vi "run.vi"() -> ()   [LabVIEW 2014]
uses:
  creeper.ctl
  nail.ctl
  block.ctl
  airplane.ctl
  <vilib>/Utility/miscctls.llb/LVPositionTypeDef.ctl
  <vilib>/Utility/inputDevices.llb/keyboardAcquire.vi
panel:
  out "step":u32
  in  "airplane":T1
  in  "Block":T2
  in  "nail":T3
  in  "creeper":T4
  out "speed":u32
  out "score":u32
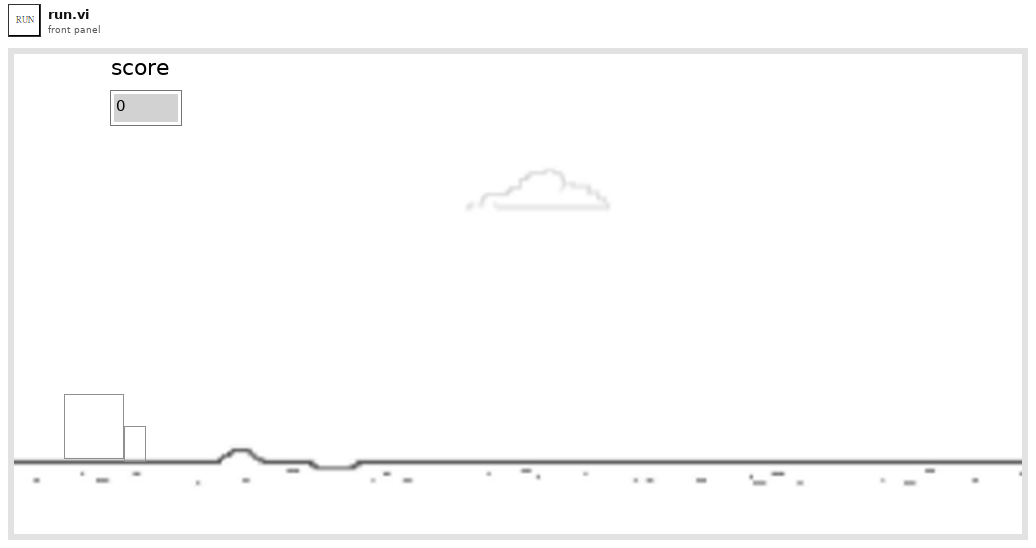
[diagram p1: front panel]
types:
  T1 = typedef "airplane.ctl" = bool
  T2 = typedef "block.ctl" = bool
  T3 = typedef "nail.ctl" = bool
  T4 = typedef "creeper.ctl" = bool
  T5 = typedef "LVPositionTypeDef.ctl" = cluster{"Left":i32, "Top":i32}
  T6 = enum16{"0", "1", "2", "3", "4", "5", "6", "7", "8", "9", "A", "B", "C", "D", "E", "F", "G", "H", "I", "J", "K", "L", "M", "N", "O", "P", "Q", "R", "S", "T", "U", "V", "W", "X", "Y", "Z", "F1", "F2", "F3", "F4", "F5", "F6", "F7", "F8", "F9", "F10", "F11", "F12", "F13", "F14", "F15", "ADD", "BACK", "BACKSLASH", "CAPITAL", "COMMA", "DECIMAL", "DELETE", "DIVIDE", "DOWN", "END", "EQUALS", "ESCAPE", "GRAVE (`)", "HOME", "INSERT", "LBRACKET", "LCONTROL", "LEFT", "L ALT", "LSHIFT", "LWIN", "MINUS", "MULTIPLY", "NEXT", "NUMLOCK", "NUMPAD_0", "NUMPAD_1", "NUMPAD_2", "NUMPAD_3", "NUMPAD_4", "NUMPAD_5", "NUMPAD_6", "NUMPAD_7", "NUMPAD_8", "NUMPAD_9", "PAUSE", "PERIOD", "PRIOR (PG UP)", "RBRACKET", "RCONTROL", "RETURN", "RIGHT", "R ALT", "RSHIFT", "RWIN", "SCROLL", "SEMICOLON", "SLASH", "SPACE", "SUBTRACT", "TAB", "UP", "ENTER (num pad)", "' (quote)"}[]
  T7 = enum16{"0", "1", "2", "3", "4", "5", "6", "7", "8", "9", "A", "B", "C", "D", "E", "F", "G", "H", "I", "J", "K", "L", "M", "N", "O", "P", "Q", "R", "S", "T", "U", "V", "W", "X", "Y", "Z", "F1", "F2", "F3", "F4", "F5", "F6", "F7", "F8", "F9", "F10", "F11", "F12", "F13", "F14", "F15", "ADD", "BACK", "BACKSLASH", "CAPITAL", "COMMA", "DECIMAL", "DELETE", "DIVIDE", "DOWN", "END", "EQUALS", "ESCAPE", "GRAVE (`)", "HOME", "INSERT", "LBRACKET", "LCONTROL", "LEFT", "L ALT", "LSHIFT", "LWIN", "MINUS", "MULTIPLY", "NEXT", "NUMLOCK", "NUMPAD_0", "NUMPAD_1", "NUMPAD_2", "NUMPAD_3", "NUMPAD_4", "NUMPAD_5", "NUMPAD_6", "NUMPAD_7", "NUMPAD_8", "NUMPAD_9", "PAUSE", "PERIOD", "PRIOR (PG UP)", "RBRACKET", "RCONTROL", "RETURN", "RIGHT", "R ALT", "RSHIFT", "RWIN", "SCROLL", "SEMICOLON", "SLASH", "SPACE", "SUBTRACT", "TAB", "UP", "ENTER (num pad)", "' (quote)"}
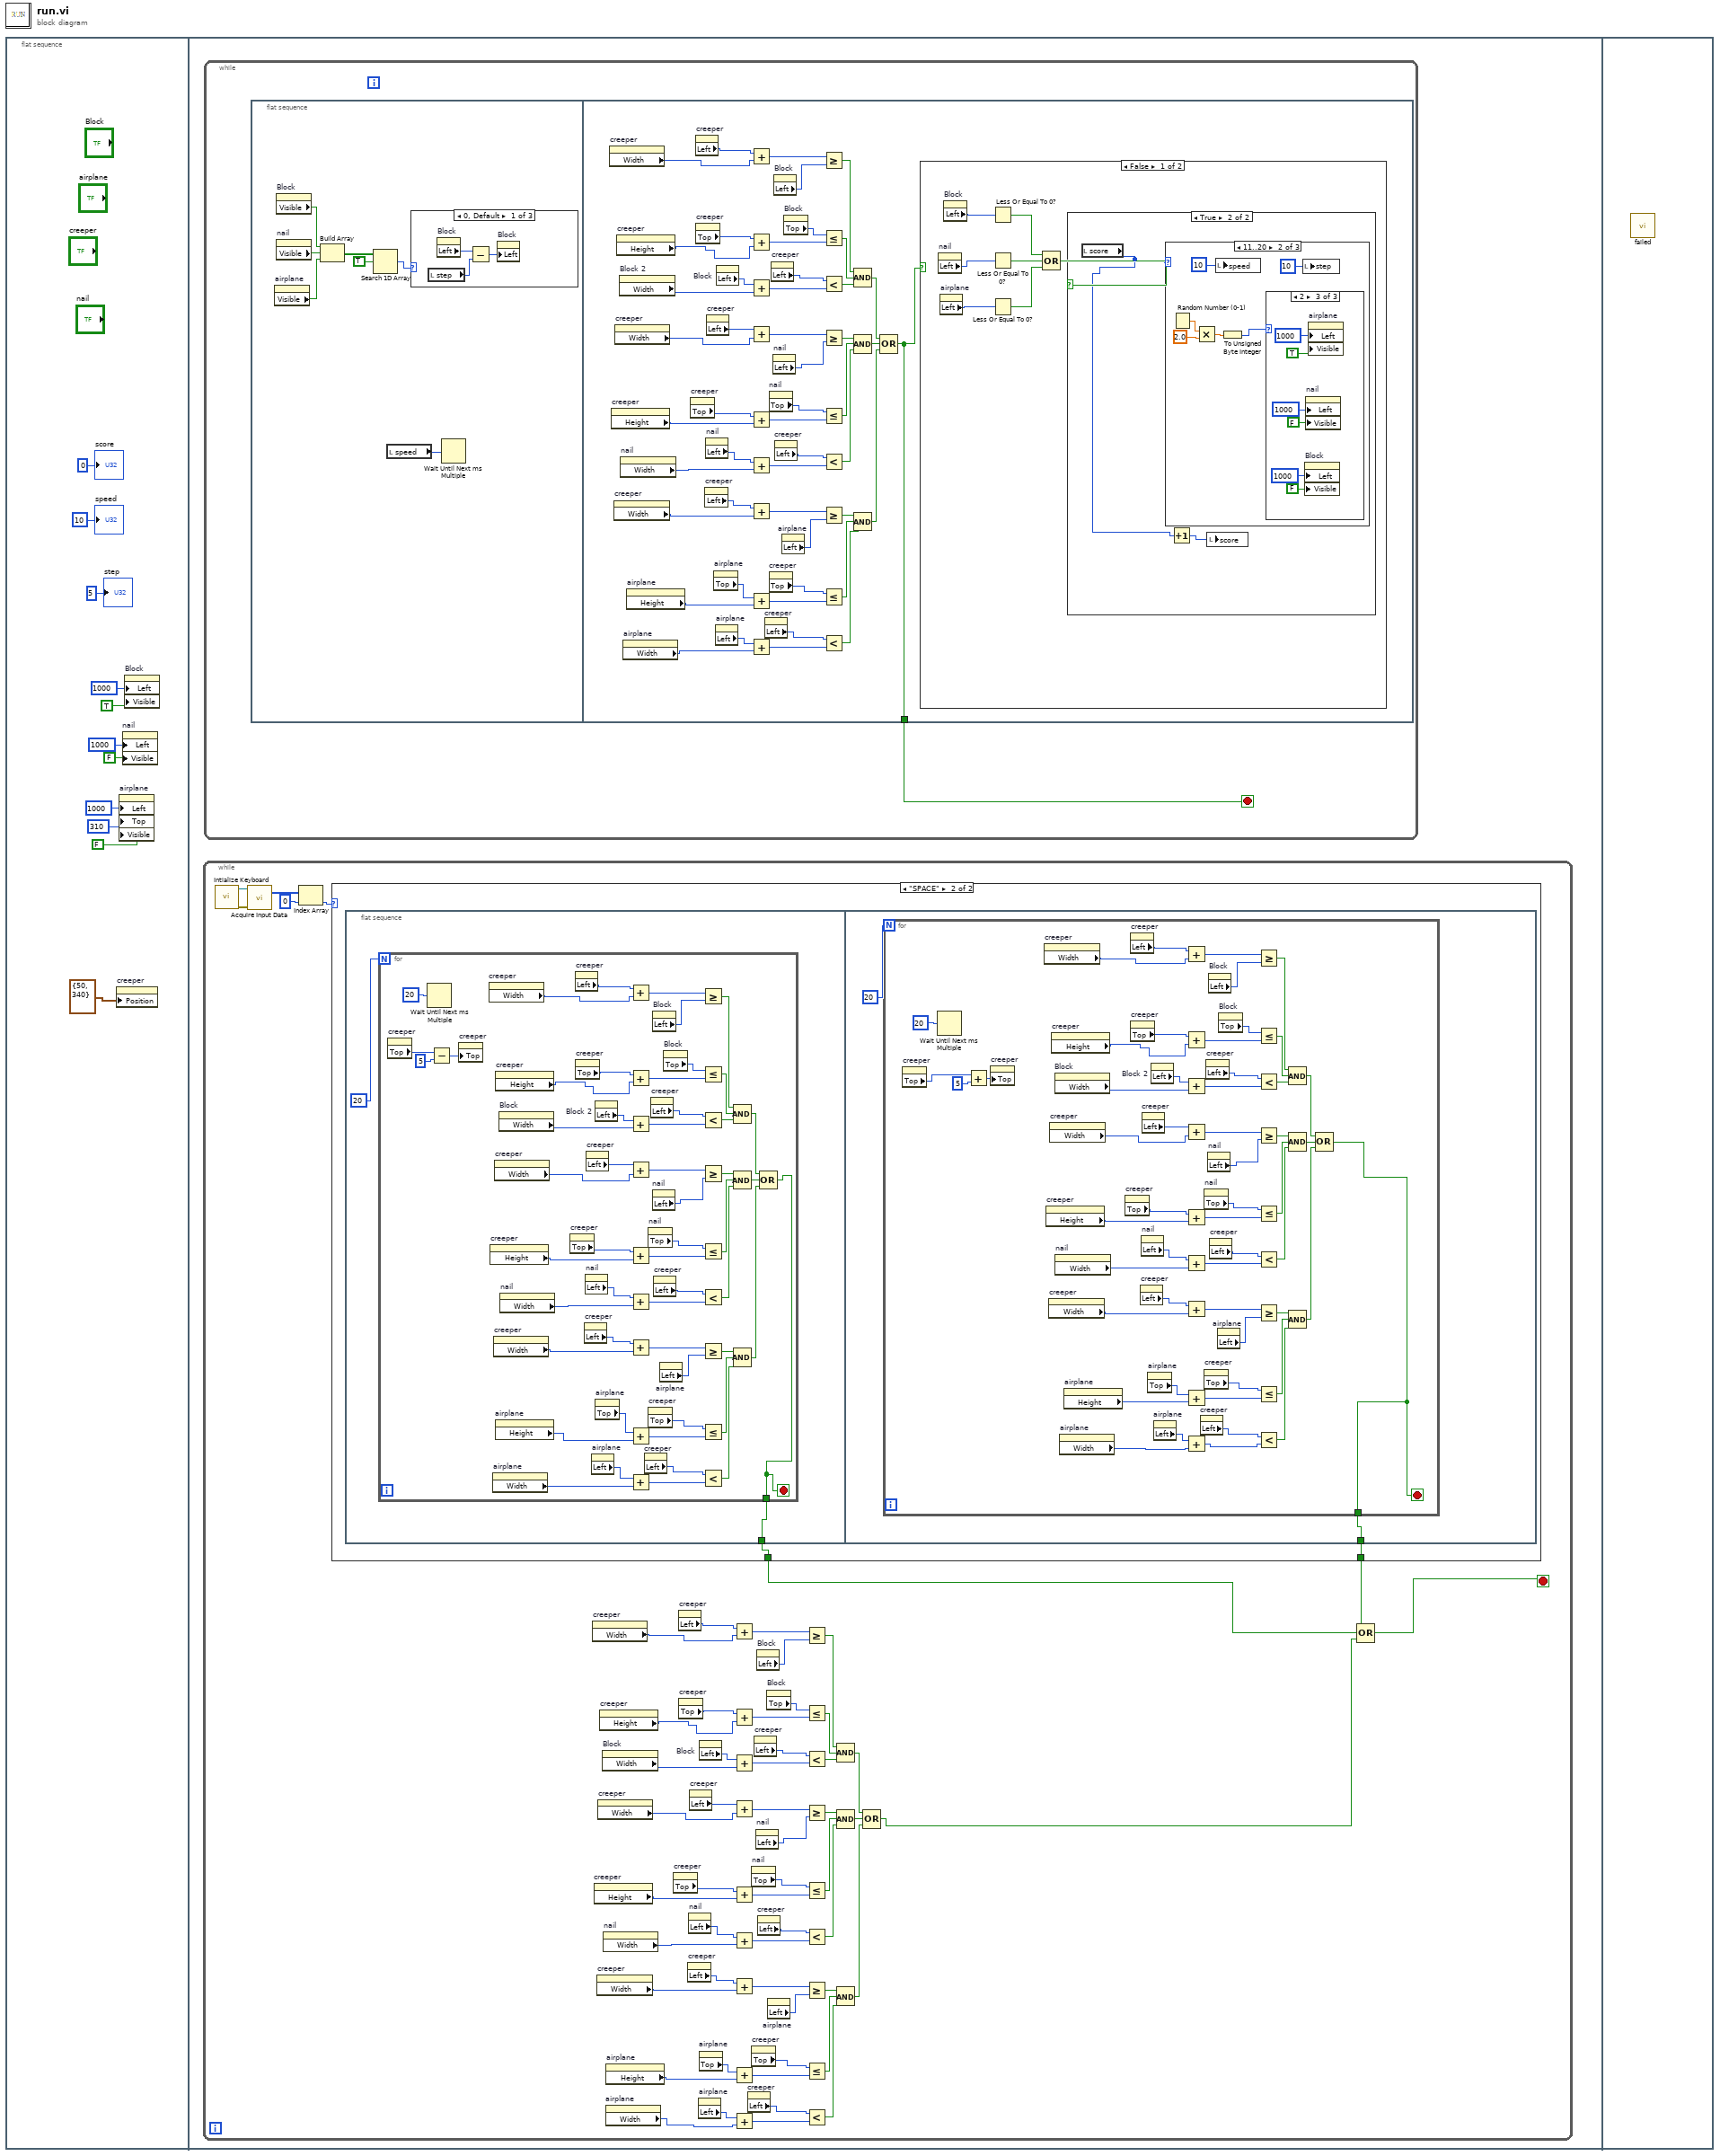
[diagram p0: block diagram]
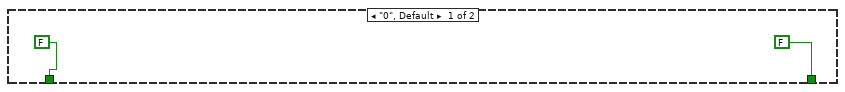
[diagram p2: hidden frame]
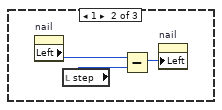
[diagram p3: hidden frame]
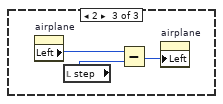
[diagram p4: hidden frame]
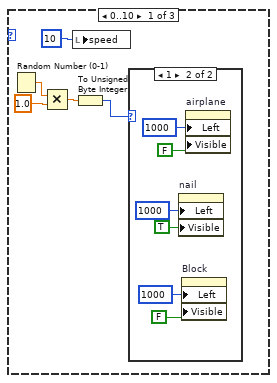
[diagram p6: hidden frame]
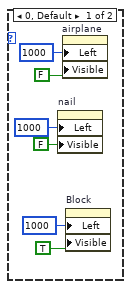
[diagram p7: hidden frame]
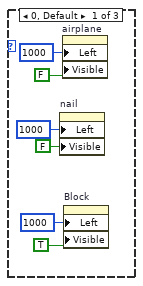
[diagram p8: hidden frame]
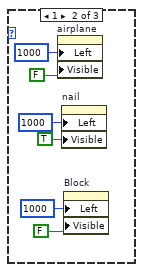
[diagram p9: hidden frame]
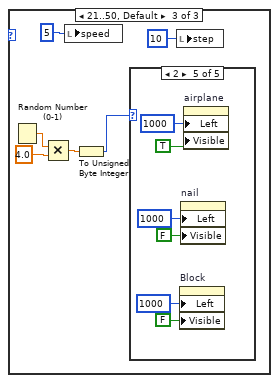
[diagram p10: hidden frame]
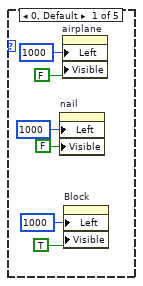
[diagram p11: hidden frame]
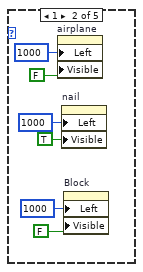
[diagram p12: hidden frame]
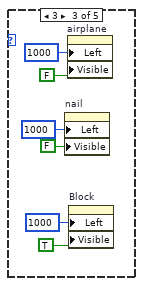
[diagram p13: hidden frame]
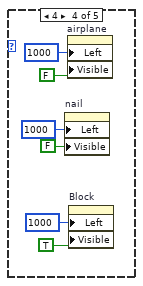
[diagram p14: hidden frame]
diagram:
  n1 = flat-sequence {
    frame #0 {
      n2 = property on="creeper" class="Bool (strict)"("Position"=T5 {"Left"=50, "Top"=340}) -> ()  [unwired: 2 in, 2 out]
      n3 = property on="airplane" class="Bool"("Left"=1000 ("Position:Left"), "Top"=310 ("Position:Top"), "Visible"=FALSE) -> ()  [unwired: 2 in, 2 out]
      n4 = property on="nail" class="Bool"("Left"=1000 ("Position:Left"), "Visible"=FALSE) -> ()  [unwired: 2 in, 2 out]
      n5 = property on="Block" class="Bool"("Left"=1000 ("Position:Left"), "Visible"=TRUE) -> ()  [unwired: 2 in, 2 out]
      "score" <- u32 0 ("score")
      "speed" <- u32 10 ("speed")
      "step" <- u32 5 ("step")
    }
    frame #1 {
      n6 = while {
        stop <- w62 stop-if-true
        n7 = call <vilib>:"Intialize Keyboard.vi"() -> ("error out"=w12:errorcluster, "device ID"=w68:refnum<k1>)  [unwired: 10 in]
        n8 = call-poly <vilib>:"Acquire Input Data.vi"("device ID"=w68, "error in (no error)"=w12) -> ("keys pressed"=w67:T6)  [unwired: 15 in, 2 out]
        n9 = Index Array(array=w67, index=0) -> (element=w65:T7)
        n10 = case shown="\"SPACE\"" w65 {
          tunnel: [FALSE w71] -> w64
          tunnel: [FALSE w72] -> w63
          frame "0", Default {
          }
          frame "SPACE" {
            n11 = flat-sequence {
              tunnel: [w73] -> w71
              tunnel: [w128] -> w72
              frame #0 {
                n12 = for {
                  N: 20 -> [_]
                  tunnel: [w80] -> w73
                  stop <- w80 stop-if-true
                  n13 = property on="creeper" class="Bool (strict)"() -> ("Top"=w125:i32)  [unwired: 2 in, 2 out]
                  n14 = Wait Until Next ms Multiple(millisecond multiple=u32 20) -> ()  [unwired: 1 out]
                  n15 = Subtract(x=w125, y=5) -> (x-y=w124:i32)
                  n16 = property on="creeper" class="Bool (strict)"("Top"=w124) -> ()  [unwired: 2 in, 2 out]
                  n17 = property on="creeper" class="Bool (strict)"() -> ("Width"=w115:u32)  [unwired: 2 in, 2 out]
                  n18 = property on="creeper" class="Bool (strict)"() -> ("Height"=w107:u32)  [unwired: 2 in, 2 out]
                  n19 = property on="airplane" class="Bool"() -> ("Width"=w76:u32)  [unwired: 2 in, 2 out]
                  n20 = property on="creeper" class="Bool (strict)"() -> ("Width"=w113:u32)  [unwired: 2 in, 2 out]
                  n21 = property on="creeper" class="Bool (strict)"() -> ("Width"=w114:u32)  [unwired: 2 in, 2 out]
                  n22 = property on="airplane" class="Bool"() -> ("Height"=w77:u32)  [unwired: 2 in, 2 out]
                  n23 = property on="creeper" class="Bool (strict)"() -> ("Height"=w103:u32)  [unwired: 2 in, 2 out]
                  n24 = property on="Block" class="Bool"() -> ("Width"=w123:u32)  [unwired: 2 in, 2 out]
                  n25 = property on="nail" class="Bool"() -> ("Width"=w119:u32)  [unwired: 2 in, 2 out]
                  n26 = property on="creeper" class="Bool (strict)"() -> ("Top"=w108:i32)  [unwired: 2 in, 2 out]
                  n27 = property on="creeper" class="Bool (strict)"() -> ("Left"=w102:i32)  [unwired: 2 in, 2 out]
                  n28 = property on="creeper" class="Bool (strict)"() -> ("Top"=w104:i32)  [unwired: 2 in, 2 out]
                  n29 = property on="creeper" class="Bool (strict)"() -> ("Left"=w110:i32)  [unwired: 2 in, 2 out]
                  n30 = property on="nail" class="Bool"() -> ("Left"=w118:i32)  [unwired: 2 in, 2 out]
                  n31 = property on="creeper" class="Bool (strict)"() -> ("Left"=w106:i32)  [unwired: 2 in, 2 out]
                  n32 = property on="airplane" class="Bool"() -> ("Left"=w75:i32)  [unwired: 2 in, 2 out]
                  n33 = property on="Block 2" class="Bool"() -> ("Left"=w122:i32)  [unwired: 2 in, 2 out]
                  n34 = property on="airplane" class="Bool"() -> ("Top"=w78:i32)  [unwired: 2 in, 2 out]
                  n35 = Add(x=w102, y=w115) -> (x+y=w81:u32)
                  n36 = Add(x=w104, y=w103) -> (x+y=w82:u32)
                  n37 = Add(x=w122, y=w123) -> (x+y=w85:u32)
                  n38 = Add(x=w106, y=w114) -> (x+y=w92:u32)
                  n39 = Add(x=w108, y=w107) -> (x+y=w91:u32)
                  n40 = Add(x=w118, y=w119) -> (x+y=w88:u32)
                  n41 = Add(x=w110, y=w113) -> (x+y=w93:u32)
                  n42 = Add(x=w78, y=w77) -> (x+y=w94:u32)
                  n43 = Add(x=w75, y=w76) -> (x+y=w95:u32)
                  n44 = property on="creeper" class="Bool (strict)"() -> ("Left"=w112:i32)  [unwired: 2 in, 2 out]
                  n45 = property on="nail" class="Bool"() -> ("Top"=w117:i32)  [unwired: 2 in, 2 out]
                  n46 = property on="creeper" class="Bool (strict)"() -> ("Top"=w111:i32)  [unwired: 2 in, 2 out]
                  n47 = property on="creeper" class="Bool (strict)"() -> ("Left"=w105:i32)  [unwired: 2 in, 2 out]
                  n48 = property on="nail" class="Bool"() -> ("Left"=w116:i32)  [unwired: 2 in, 2 out]
                  n49 = property on="Block" class="Bool"() -> ("Left"=w120:i32)  [unwired: 2 in, 2 out]
                  n50 = property on="creeper" class="Bool (strict)"() -> ("Left"=w109:i32)  [unwired: 2 in, 2 out]
                  n51 = property on="airplane" class="Bool"() -> ("Left"=w79:i32)  [unwired: 2 in, 2 out]
                  n52 = property on="Block" class="Bool"() -> ("Top"=w121:i32)  [unwired: 2 in, 2 out]
                  n53 = Greater Or Equal?(x=w81, y=w120) -> (x >= y?=w83:bool)
                  n54 = Less Or Equal?(x=w121, y=w82) -> (x <= y?=w84:bool)
                  n55 = Less?(x=w105, y=w85) -> (x < y?=w86:bool)
                  n56 = Greater Or Equal?(x=w92, y=w116) -> (x >= y?=w90:bool)
                  n57 = Less Or Equal?(x=w117, y=w91) -> (x <= y?=w89:bool)
                  n58 = Less?(x=w109, y=w88) -> (x < y?=w87:bool)
                  n59 = Greater Or Equal?(x=w93, y=w79) -> (x >= y?=w96:bool)
                  n60 = Less Or Equal?(x=w111, y=w94) -> (x <= y?=w97:bool)
                  n61 = Less?(x=w112, y=w95) -> (x < y?=w98:bool)
                  n62 = Compound Arithmetic op=AND(w83, w84, w86) -> (w99:bool)
                  n63 = Compound Arithmetic op=AND(w90, w89, w87) -> (w100:bool)
                  n64 = Compound Arithmetic op=AND(w96, w97, w98) -> (w101:bool)
                  n65 = Compound Arithmetic op=OR(w99, w100, w101) -> (w80:bool)
                }
              }
              frame #1 {
                n66 = for {
                  N: 20 -> [_]
                  tunnel: [w136] -> w128
                  stop <- w136 stop-if-true
                  n67 = property on="creeper" class="Bool (strict)"() -> ("Top"=w180:i32)  [unwired: 2 in, 2 out]
                  n68 = Wait Until Next ms Multiple(millisecond multiple=u32 20) -> ()  [unwired: 1 out]
                  n69 = Add(x=w180, y=5) -> (x+y=w179:i32)
                  n70 = property on="creeper" class="Bool (strict)"("Top"=w179) -> ()  [unwired: 2 in, 2 out]
                  n71 = property on="creeper" class="Bool (strict)"() -> ("Width"=w145:u32)  [unwired: 2 in, 2 out]
                  n72 = property on="creeper" class="Bool (strict)"() -> ("Height"=w153:u32)  [unwired: 2 in, 2 out]
                  n73 = property on="creeper" class="Bool (strict)"() -> ("Width"=w147:u32)  [unwired: 2 in, 2 out]
                  n74 = property on="creeper" class="Bool (strict)"() -> ("Width"=w146:u32)  [unwired: 2 in, 2 out]
                  n75 = property on="creeper" class="Bool (strict)"() -> ("Height"=w157:u32)  [unwired: 2 in, 2 out]
                  n76 = property on="Block" class="Bool"() -> ("Width"=w137:u32)  [unwired: 2 in, 2 out]
                  n77 = property on="nail" class="Bool"() -> ("Width"=w141:u32)  [unwired: 2 in, 2 out]
                  n78 = property on="airplane" class="Bool"() -> ("Width"=w131:u32)  [unwired: 2 in, 2 out]
                  n79 = property on="airplane" class="Bool"() -> ("Height"=w132:u32)  [unwired: 2 in, 2 out]
                  n80 = property on="creeper" class="Bool (strict)"() -> ("Top"=w152:i32)  [unwired: 2 in, 2 out]
                  n81 = property on="creeper" class="Bool (strict)"() -> ("Left"=w158:i32)  [unwired: 2 in, 2 out]
                  n82 = property on="creeper" class="Bool (strict)"() -> ("Top"=w156:i32)  [unwired: 2 in, 2 out]
                  n83 = property on="creeper" class="Bool (strict)"() -> ("Left"=w150:i32)  [unwired: 2 in, 2 out]
                  n84 = property on="nail" class="Bool"() -> ("Left"=w142:i32)  [unwired: 2 in, 2 out]
                  n85 = property on="creeper" class="Bool (strict)"() -> ("Left"=w154:i32)  [unwired: 2 in, 2 out]
                  n86 = property on="airplane" class="Bool"() -> ("Top"=w133:i32)  [unwired: 2 in, 2 out]
                  n87 = property on="Block 2" class="Bool"() -> ("Left"=w138:i32)  [unwired: 2 in, 2 out]
                  n88 = property on="airplane" class="Bool"() -> ("Left"=w130:i32)  [unwired: 2 in, 2 out]
                  n89 = Add(x=w158, y=w145) -> (x+y=w178:u32)
                  n90 = Add(x=w156, y=w157) -> (x+y=w177:u32)
                  n91 = Add(x=w138, y=w137) -> (x+y=w174:u32)
                  n92 = Add(x=w154, y=w146) -> (x+y=w167:u32)
                  n93 = Add(x=w152, y=w153) -> (x+y=w168:u32)
                  n94 = Add(x=w142, y=w141) -> (x+y=w171:u32)
                  n95 = Add(x=w150, y=w147) -> (x+y=w166:u32)
                  n96 = Add(x=w133, y=w132) -> (x+y=w165:u32)
                  n97 = Add(x=w130, y=w131) -> (x+y=w135:u32)
                  n98 = property on="creeper" class="Bool (strict)"() -> ("Left"=w148:i32)  [unwired: 2 in, 2 out]
                  n99 = property on="nail" class="Bool"() -> ("Top"=w143:i32)  [unwired: 2 in, 2 out]
                  n100 = property on="creeper" class="Bool (strict)"() -> ("Top"=w149:i32)  [unwired: 2 in, 2 out]
                  n101 = property on="creeper" class="Bool (strict)"() -> ("Left"=w155:i32)  [unwired: 2 in, 2 out]
                  n102 = property on="nail" class="Bool"() -> ("Left"=w144:i32)  [unwired: 2 in, 2 out]
                  n103 = property on="Block" class="Bool"() -> ("Left"=w140:i32)  [unwired: 2 in, 2 out]
                  n104 = property on="creeper" class="Bool (strict)"() -> ("Left"=w151:i32)  [unwired: 2 in, 2 out]
                  n105 = property on="airplane" class="Bool"() -> ("Left"=w134:i32)  [unwired: 2 in, 2 out]
                  n106 = property on="Block" class="Bool"() -> ("Top"=w139:i32)  [unwired: 2 in, 2 out]
                  n107 = Greater Or Equal?(x=w178, y=w140) -> (x >= y?=w176:bool)
                  n108 = Less Or Equal?(x=w139, y=w177) -> (x <= y?=w175:bool)
                  n109 = Less?(x=w155, y=w174) -> (x < y?=w173:bool)
                  n110 = Greater Or Equal?(x=w167, y=w144) -> (x >= y?=w169:bool)
                  n111 = Less Or Equal?(x=w143, y=w168) -> (x <= y?=w170:bool)
                  n112 = Less?(x=w151, y=w171) -> (x < y?=w172:bool)
                  n113 = Greater Or Equal?(x=w166, y=w134) -> (x >= y?=w164:bool)
                  n114 = Less Or Equal?(x=w149, y=w165) -> (x <= y?=w163:bool)
                  n115 = Less?(x=w148, y=w135) -> (x < y?=w162:bool)
                  n116 = Compound Arithmetic op=AND(w176, w175, w173) -> (w161:bool)
                  n117 = Compound Arithmetic op=AND(w169, w170, w172) -> (w160:bool)
                  n118 = Compound Arithmetic op=AND(w164, w163, w162) -> (w159:bool)
                  n119 = Compound Arithmetic op=OR(w161, w160, w159) -> (w136:bool)
                }
              }
            }
          }
        }
        n120 = property on="creeper" class="Bool (strict)"() -> ("Width"=w53:u32)  [unwired: 2 in, 2 out]
        n121 = property on="creeper" class="Bool (strict)"() -> ("Height"=w45:u32)  [unwired: 2 in, 2 out]
        n122 = property on="creeper" class="Bool (strict)"() -> ("Width"=w51:u32)  [unwired: 2 in, 2 out]
        n123 = property on="creeper" class="Bool (strict)"() -> ("Width"=w52:u32)  [unwired: 2 in, 2 out]
        n124 = property on="creeper" class="Bool (strict)"() -> ("Height"=w41:u32)  [unwired: 2 in, 2 out]
        n125 = property on="Block" class="Bool"() -> ("Width"=w61:u32)  [unwired: 2 in, 2 out]
        n126 = property on="nail" class="Bool"() -> ("Width"=w57:u32)  [unwired: 2 in, 2 out]
        n127 = property on="airplane" class="Bool"() -> ("Width"=w14:u32)  [unwired: 2 in, 2 out]
        n128 = property on="airplane" class="Bool"() -> ("Height"=w15:u32)  [unwired: 2 in, 2 out]
        n129 = property on="creeper" class="Bool (strict)"() -> ("Top"=w46:i32)  [unwired: 2 in, 2 out]
        n130 = property on="creeper" class="Bool (strict)"() -> ("Left"=w40:i32)  [unwired: 2 in, 2 out]
        n131 = property on="creeper" class="Bool (strict)"() -> ("Top"=w42:i32)  [unwired: 2 in, 2 out]
        n132 = property on="creeper" class="Bool (strict)"() -> ("Left"=w48:i32)  [unwired: 2 in, 2 out]
        n133 = property on="nail" class="Bool"() -> ("Left"=w56:i32)  [unwired: 2 in, 2 out]
        n134 = property on="creeper" class="Bool (strict)"() -> ("Left"=w44:i32)  [unwired: 2 in, 2 out]
        n135 = property on="airplane" class="Bool"() -> ("Left"=w13:i32)  [unwired: 2 in, 2 out]
        n136 = property on="Block" class="Bool"() -> ("Left"=w60:i32)  [unwired: 2 in, 2 out]
        n137 = property on="airplane" class="Bool"() -> ("Top"=w16:i32)  [unwired: 2 in, 2 out]
        n138 = Add(x=w40, y=w53) -> (x+y=w20:u32)
        n139 = Add(x=w42, y=w41) -> (x+y=w21:u32)
        n140 = Add(x=w60, y=w61) -> (x+y=w24:u32)
        n141 = Add(x=w44, y=w52) -> (x+y=w31:u32)
        n142 = Add(x=w46, y=w45) -> (x+y=w30:u32)
        n143 = Add(x=w56, y=w57) -> (x+y=w27:u32)
        n144 = Add(x=w48, y=w51) -> (x+y=w32:u32)
        n145 = Add(x=w16, y=w15) -> (x+y=w33:u32)
        n146 = Add(x=w13, y=w14) -> (x+y=w18:u32)
        n147 = property on="creeper" class="Bool (strict)"() -> ("Left"=w50:i32)  [unwired: 2 in, 2 out]
        n148 = property on="nail" class="Bool"() -> ("Top"=w55:i32)  [unwired: 2 in, 2 out]
        n149 = property on="creeper" class="Bool (strict)"() -> ("Top"=w49:i32)  [unwired: 2 in, 2 out]
        n150 = property on="creeper" class="Bool (strict)"() -> ("Left"=w43:i32)  [unwired: 2 in, 2 out]
        n151 = property on="nail" class="Bool"() -> ("Left"=w54:i32)  [unwired: 2 in, 2 out]
        n152 = property on="Block" class="Bool"() -> ("Left"=w58:i32)  [unwired: 2 in, 2 out]
        n153 = property on="creeper" class="Bool (strict)"() -> ("Left"=w47:i32)  [unwired: 2 in, 2 out]
        n154 = property on="Block" class="Bool"() -> ("Top"=w59:i32)  [unwired: 2 in, 2 out]
        n155 = property on="airplane" class="Bool"() -> ("Left"=w17:i32)  [unwired: 2 in, 2 out]
        n156 = Greater Or Equal?(x=w20, y=w58) -> (x >= y?=w22:bool)
        n157 = Less Or Equal?(x=w59, y=w21) -> (x <= y?=w23:bool)
        n158 = Less?(x=w43, y=w24) -> (x < y?=w25:bool)
        n159 = Greater Or Equal?(x=w31, y=w54) -> (x >= y?=w29:bool)
        n160 = Less Or Equal?(x=w55, y=w30) -> (x <= y?=w28:bool)
        n161 = Less?(x=w47, y=w27) -> (x < y?=w26:bool)
        n162 = Greater Or Equal?(x=w32, y=w17) -> (x >= y?=w34:bool)
        n163 = Less Or Equal?(x=w49, y=w33) -> (x <= y?=w35:bool)
        n164 = Less?(x=w50, y=w18) -> (x < y?=w36:bool)
        n165 = Compound Arithmetic op=AND(w22, w23, w25) -> (w37:bool)
        n166 = Compound Arithmetic op=AND(w29, w28, w26) -> (w38:bool)
        n167 = Compound Arithmetic op=AND(w34, w35, w36) -> (w39:bool)
        n168 = Compound Arithmetic op=OR(w37, w38, w39) -> (w19:bool)
        n169 = Compound Arithmetic op=OR(w63, w64, w19) -> (w62:bool)
      }
      n170 = while {
        stop <- w183 stop-if-true
        n171 = flat-sequence {
          tunnel: [w227] -> w183
          frame #0 {
            n172 = property on="airplane" class="Bool"() -> ("Visible"=w184:bool)  [unwired: 2 in, 2 out]
            n173 = property on="Block" class="Bool"() -> ("Visible"=w185:bool)  [unwired: 2 in, 2 out]
            n174 = property on="nail" class="Bool"() -> ("Visible"=w186:bool)  [unwired: 2 in, 2 out]
            n175 = Build Array(w185, w186, w184) -> (w190:bool[])
            n176 = Search 1D Array(1D array=w190, element=TRUE) -> (index of element=w189:i32)  [unwired: 1 in]
            n177 = local read "speed"() -> (w187:u32)
            n178 = case shown="0, Default" w189 {
              frame 0, Default {
                n179 = local read "step"() -> (w191:u32)
                n180 = property on="Block" class="Bool"() -> ("Left"=w193:i32)  [unwired: 2 in, 2 out]
                n181 = Subtract(x=w193, y=w191) -> (x-y=w192:u32)
                n182 = property on="Block" class="Bool"("Left"=w192) -> ()  [unwired: 2 in, 2 out]
              }
              frame 1 {
                n183 = property on="nail" class="Bool"() -> ("Left"=w196:i32)  [unwired: 2 in, 2 out]
                n184 = local read "step"() -> (w194:u32)
                n185 = Subtract(x=w196, y=w194) -> (x-y=w195:u32)
                n186 = property on="nail" class="Bool"("Left"=w195) -> ()  [unwired: 2 in, 2 out]
              }
              frame 2 {
                n187 = property on="airplane" class="Bool"() -> ("Left"=w199:i32)  [unwired: 2 in, 2 out]
                n188 = local read "step"() -> (w197:u32)
                n189 = Subtract(x=w199, y=w197) -> (x-y=w198:u32)
                n190 = property on="airplane" class="Bool"("Left"=w198) -> ()  [unwired: 2 in, 2 out]
              }
            }
            n191 = Wait Until Next ms Multiple(millisecond multiple=w187) -> ()  [unwired: 1 out]
          }
          frame #1 {
            n192 = property on="creeper" class="Bool (strict)"() -> ("Width"=w213:u32)  [unwired: 2 in, 2 out]
            n193 = property on="creeper" class="Bool (strict)"() -> ("Height"=w221:u32)  [unwired: 2 in, 2 out]
            n194 = property on="creeper" class="Bool (strict)"() -> ("Width"=w215:u32)  [unwired: 2 in, 2 out]
            n195 = property on="creeper" class="Bool (strict)"() -> ("Width"=w214:u32)  [unwired: 2 in, 2 out]
            n196 = property on="creeper" class="Bool (strict)"() -> ("Height"=w225:u32)  [unwired: 2 in, 2 out]
            n197 = property on="Block 2" class="Bool"() -> ("Width"=w205:u32)  [unwired: 2 in, 2 out]
            n198 = property on="nail" class="Bool"() -> ("Width"=w209:u32)  [unwired: 2 in, 2 out]
            n199 = property on="airplane" class="Bool"() -> ("Width"=w201:u32)  [unwired: 2 in, 2 out]
            n200 = property on="airplane" class="Bool"() -> ("Height"=w202:u32)  [unwired: 2 in, 2 out]
            n201 = property on="creeper" class="Bool (strict)"() -> ("Top"=w220:i32)  [unwired: 2 in, 2 out]
            n202 = property on="creeper" class="Bool (strict)"() -> ("Left"=w226:i32)  [unwired: 2 in, 2 out]
            n203 = property on="creeper" class="Bool (strict)"() -> ("Top"=w224:i32)  [unwired: 2 in, 2 out]
            n204 = property on="creeper" class="Bool (strict)"() -> ("Left"=w218:i32)  [unwired: 2 in, 2 out]
            n205 = property on="nail" class="Bool"() -> ("Left"=w210:i32)  [unwired: 2 in, 2 out]
            n206 = property on="creeper" class="Bool (strict)"() -> ("Left"=w222:i32)  [unwired: 2 in, 2 out]
            n207 = property on="airplane" class="Bool"() -> ("Top"=w203:i32)  [unwired: 2 in, 2 out]
            n208 = property on="airplane" class="Bool"() -> ("Left"=w200:i32)  [unwired: 2 in, 2 out]
            n209 = property on="Block" class="Bool"() -> ("Left"=w206:i32)  [unwired: 2 in, 2 out]
            n210 = Add(x=w226, y=w213) -> (x+y=w248:u32)
            n211 = Add(x=w224, y=w225) -> (x+y=w247:u32)
            n212 = Add(x=w206, y=w205) -> (x+y=w244:u32)
            n213 = Add(x=w222, y=w214) -> (x+y=w237:u32)
            n214 = Add(x=w220, y=w221) -> (x+y=w238:u32)
            n215 = Add(x=w210, y=w209) -> (x+y=w241:u32)
            n216 = Add(x=w218, y=w215) -> (x+y=w236:u32)
            n217 = Add(x=w203, y=w202) -> (x+y=w235:u32)
            n218 = Add(x=w200, y=w201) -> (x+y=w234:u32)
            n219 = property on="creeper" class="Bool (strict)"() -> ("Left"=w216:i32)  [unwired: 2 in, 2 out]
            n220 = property on="nail" class="Bool"() -> ("Top"=w211:i32)  [unwired: 2 in, 2 out]
            n221 = property on="creeper" class="Bool (strict)"() -> ("Top"=w217:i32)  [unwired: 2 in, 2 out]
            n222 = property on="creeper" class="Bool (strict)"() -> ("Left"=w223:i32)  [unwired: 2 in, 2 out]
            n223 = property on="nail" class="Bool"() -> ("Left"=w212:i32)  [unwired: 2 in, 2 out]
            n224 = property on="Block" class="Bool"() -> ("Left"=w208:i32)  [unwired: 2 in, 2 out]
            n225 = property on="creeper" class="Bool (strict)"() -> ("Left"=w219:i32)  [unwired: 2 in, 2 out]
            n226 = property on="airplane" class="Bool"() -> ("Left"=w204:i32)  [unwired: 2 in, 2 out]
            n227 = property on="Block" class="Bool"() -> ("Top"=w207:i32)  [unwired: 2 in, 2 out]
            n228 = Greater Or Equal?(x=w248, y=w208) -> (x >= y?=w246:bool)
            n229 = Less Or Equal?(x=w207, y=w247) -> (x <= y?=w245:bool)
            n230 = Less?(x=w223, y=w244) -> (x < y?=w243:bool)
            n231 = Greater Or Equal?(x=w237, y=w212) -> (x >= y?=w239:bool)
            n232 = Less Or Equal?(x=w211, y=w238) -> (x <= y?=w240:bool)
            n233 = Less?(x=w219, y=w241) -> (x < y?=w242:bool)
            n234 = Greater Or Equal?(x=w236, y=w204) -> (x >= y?=w233:bool)
            n235 = Less Or Equal?(x=w217, y=w235) -> (x <= y?=w232:bool)
            n236 = Less?(x=w216, y=w234) -> (x < y?=w231:bool)
            n237 = Compound Arithmetic op=AND(w246, w245, w243) -> (w230:bool)
            n238 = Compound Arithmetic op=AND(w239, w240, w242) -> (w229:bool)
            n239 = Compound Arithmetic op=AND(w233, w232, w231) -> (w228:bool)
            n240 = Compound Arithmetic op=OR(w230, w229, w228) -> (w227:bool)
            n241 = case shown="False" w227 {
              frame False {
                n242 = property on="nail" class="Bool"() -> ("Left"=w251:i32)  [unwired: 2 in, 2 out]
                n243 = property on="airplane" class="Bool"() -> ("Left"=w249:i32)  [unwired: 2 in, 2 out]
                n244 = property on="Block" class="Bool"() -> ("Left"=w250:i32)  [unwired: 2 in, 2 out]
                n245 = Less Or Equal To 0?(x=w250) -> (x <= 0?=w255:bool)
                n246 = Less Or Equal To 0?(x=w251) -> (x <= 0?=w254:bool)
                n247 = Less Or Equal To 0?(x=w249) -> (x <= 0?=w253:bool)
                n248 = Compound Arithmetic op=OR(w255, w254, w253) -> (w252:bool)
                n249 = case shown="True" w252 {
                  frame False {
                  }
                  frame True {
                    n250 = local read "score"() -> (w256:u32)
                    n251 = case shown="11..20" w256 {
                      frame 0..10 {
                        n252 = Random Number (0-1)() -> (number: 0 to 1=w258:dbl)
                        n253 = Multiply(x=w258, y=1.0) -> (x*y=w260:dbl)
                        n254 = local write "speed"(u32 10 ("speed")) -> ()
                        n255 = To Unsigned Byte Integer(number=w260) -> (unsigned 8bit integer=w261:u8)
                        n256 = case shown="1" w261 {
                          frame 0, Default {
                            n257 = property on="nail" class="Bool"("Left"=1000 ("Position:Left"), "Visible"=FALSE) -> ()  [unwired: 2 in, 2 out]
                            n258 = property on="airplane" class="Bool"("Left"=1000 ("Position:Left"), "Visible"=FALSE) -> ()  [unwired: 2 in, 2 out]
                            n259 = property on="Block" class="Bool"("Left"=1000 ("Position:Left"), "Visible"=TRUE) -> ()  [unwired: 2 in, 2 out]
                          }
                          frame 1 {
                            n260 = property on="nail" class="Bool"("Left"=1000 ("Position:Left"), "Visible"=TRUE) -> ()  [unwired: 2 in, 2 out]
                            n261 = property on="Block" class="Bool"("Left"=1000 ("Position:Left"), "Visible"=FALSE) -> ()  [unwired: 2 in, 2 out]
                            n262 = property on="airplane" class="Bool"("Left"=1000 ("Position:Left"), "Visible"=FALSE) -> ()  [unwired: 2 in, 2 out]
                          }
                        }
                      }
                      frame 11..20 {
                        n263 = Random Number (0-1)() -> (number: 0 to 1=w276:dbl)
                        n264 = Multiply(x=w276, y=2.0) -> (x*y=w278:dbl)
                        n265 = local write "speed"(u32 10 ("speed")) -> ()
                        n266 = To Unsigned Byte Integer(number=w278) -> (unsigned 8bit integer=w279:u8)
                        n267 = case shown="2" w279 {
                          frame 0, Default {
                            n268 = property on="nail" class="Bool"("Left"=1000 ("Position:Left"), "Visible"=FALSE) -> ()  [unwired: 2 in, 2 out]
                            n269 = property on="airplane" class="Bool"("Left"=1000 ("Position:Left"), "Visible"=FALSE) -> ()  [unwired: 2 in, 2 out]
                            n270 = property on="Block" class="Bool"("Left"=1000 ("Position:Left"), "Visible"=TRUE) -> ()  [unwired: 2 in, 2 out]
                          }
                          frame 1 {
                            n271 = property on="airplane" class="Bool"("Left"=1000 ("Position:Left"), "Visible"=FALSE) -> ()  [unwired: 2 in, 2 out]
                            n272 = property on="nail" class="Bool"("Left"=1000 ("Position:Left"), "Visible"=TRUE) -> ()  [unwired: 2 in, 2 out]
                            n273 = property on="Block" class="Bool"("Left"=1000 ("Position:Left"), "Visible"=FALSE) -> ()  [unwired: 2 in, 2 out]
                          }
                          frame 2 {
                            n274 = property on="Block" class="Bool"("Left"=1000 ("Position:Left"), "Visible"=FALSE) -> ()  [unwired: 2 in, 2 out]
                            n275 = property on="nail" class="Bool"("Left"=1000 ("Position:Left"), "Visible"=FALSE) -> ()  [unwired: 2 in, 2 out]
                            n276 = property on="airplane" class="Bool"("Left"=1000 ("Position:Left"), "Visible"=TRUE) -> ()  [unwired: 2 in, 2 out]
                          }
                        }
                        n277 = local write "step"(u32 10 ("step")) -> ()
                      }
                      frame 21..50, Default {
                        n278 = Random Number (0-1)() -> (number: 0 to 1=w300:dbl)
                        n279 = Multiply(x=w300, y=4.0) -> (x*y=w302:dbl)
                        n280 = local write "speed"(u32 5 ("speed")) -> ()
                        n281 = To Unsigned Byte Integer(number=w302) -> (unsigned 8bit integer=w303:u8)
                        n282 = case shown="2" w303 {
                          frame 0, Default {
                            n283 = property on="nail" class="Bool"("Left"=1000 ("Position:Left"), "Visible"=FALSE) -> ()  [unwired: 2 in, 2 out]
                            n284 = property on="airplane" class="Bool"("Left"=1000 ("Position:Left"), "Visible"=FALSE) -> ()  [unwired: 2 in, 2 out]
                            n285 = property on="Block" class="Bool"("Left"=1000 ("Position:Left"), "Visible"=TRUE) -> ()  [unwired: 2 in, 2 out]
                          }
                          frame 1 {
                            n286 = property on="airplane" class="Bool"("Left"=1000 ("Position:Left"), "Visible"=FALSE) -> ()  [unwired: 2 in, 2 out]
                            n287 = property on="nail" class="Bool"("Left"=1000 ("Position:Left"), "Visible"=TRUE) -> ()  [unwired: 2 in, 2 out]
                            n288 = property on="Block" class="Bool"("Left"=1000 ("Position:Left"), "Visible"=FALSE) -> ()  [unwired: 2 in, 2 out]
                          }
                          frame 3 {
                            n289 = property on="nail" class="Bool"("Left"=1000 ("Position:Left"), "Visible"=FALSE) -> ()  [unwired: 2 in, 2 out]
                            n290 = property on="airplane" class="Bool"("Left"=1000 ("Position:Left"), "Visible"=FALSE) -> ()  [unwired: 2 in, 2 out]
                            n291 = property on="Block" class="Bool"("Left"=1000 ("Position:Left"), "Visible"=TRUE) -> ()  [unwired: 2 in, 2 out]
                          }
                          frame 4 {
                            n292 = property on="nail" class="Bool"("Left"=1000 ("Position:Left"), "Visible"=FALSE) -> ()  [unwired: 2 in, 2 out]
                            n293 = property on="airplane" class="Bool"("Left"=1000 ("Position:Left"), "Visible"=FALSE) -> ()  [unwired: 2 in, 2 out]
                            n294 = property on="Block" class="Bool"("Left"=1000 ("Position:Left"), "Visible"=TRUE) -> ()  [unwired: 2 in, 2 out]
                          }
                          frame 2 {
                            n295 = property on="Block" class="Bool"("Left"=1000 ("Position:Left"), "Visible"=FALSE) -> ()  [unwired: 2 in, 2 out]
                            n296 = property on="nail" class="Bool"("Left"=1000 ("Position:Left"), "Visible"=FALSE) -> ()  [unwired: 2 in, 2 out]
                            n297 = property on="airplane" class="Bool"("Left"=1000 ("Position:Left"), "Visible"=TRUE) -> ()  [unwired: 2 in, 2 out]
                          }
                        }
                        n298 = local write "step"(u32 10 ("step")) -> ()
                      }
                    }
                    n299 = Increment(x=w256) -> (x+1=w257:u32)
                    n300 = local write "score"(w257) -> ()
                  }
                }
              }
              frame True {
              }
            }
          }
        }
      }
    }
    frame #2 {
      n301 = call "failed.vi"() -> ()  [unwired: 12 in]
    }
  }
